vi "Teleop.vi"(10 "Match Info":T1={"Autonomous Elapsed Seconds"=0.0, "TeleOp Elapsed Seconds"=0.0, "Disabled Elapsed Seconds"=0.0, "Visited Autonomous"=FALSE, "Visited TeleOp"=FALSE, "Visited Disabled"=FALSE, "Autonomous Settings"={"Autonomous Style"=enum."Independent", "VI Refnum"=refnum}}, 11 "Call Context":T2) -> ()   [LabVIEW 2011]
doc: "This VI is called for each TeleOp packet received from the DS where the robot is not disabled. It is often used to read from the joysticks and update I/O or to update setpoints for timed control loops. It should complete and return within 20 milliseconds or it may miss DS packets."
uses:
  <vilib>/Rock Robotics/WPI/DriverStation/WPI_DriverStationDerivedRobotMode.ctl
  <vilib>/Rock Robotics/WPI/DriverStation/WPI_DriverStationMatch Info.ctl
  Robot Global Data.vi
  <vilib>/Rock Robotics/WPI/Solenoid/Deprecated/WPI_SolenoidSetBool.vi
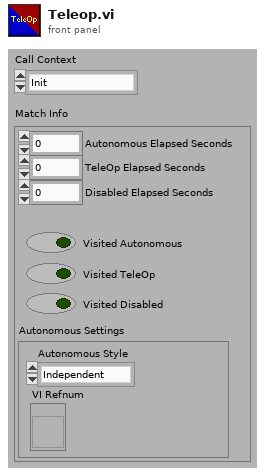
[diagram p1: front panel]
types:
  T1 = typedef "WPI_DriverStationMatch Info.ctl" = cluster{"Autonomous Elapsed Seconds":dbl, "TeleOp Elapsed Seconds":dbl, "Disabled Elapsed Seconds":dbl, "Visited Autonomous":bool, "Visited TeleOp":bool, "Visited Disabled":bool, "Autonomous Settings":cluster{"Autonomous Style":enum16{"Iterative", "Independent"}, "VI Refnum":refnum<vi>}}
  T2 = typedef "WPI_DriverStationDerivedRobotMode.ctl" = enum16{"Init", "Execute", "Stop"}
  T3 = typedef "WPI_DigitalInputDevRef.ctl" = cluster{"DevStatus":errorcluster, "DIO Channel":T4, "Digital Module":T5}
  T4 = typedef "FPGA_DIOChannel.ctl" = enum8{"DIO 1", "DIO 2", "DIO 3", "DIO 4", "DIO 5", "DIO 6", "DIO 7", "DIO 8", "DIO 9", "DIO 10", "DIO 11", "DIO 12", "DIO 13", "DIO 14", "Invalid"}
  T5 = typedef "FPGA_TypedefDigitalModule.ctl" = enum16{"Digital Module 1", "Digital Module 2"}
  T6 = typedef "WPI_ServoDeviceRef.ctl" = cluster{"DeviceStatus":errorcluster, "Digital Module":T5, "PWM Channel":T7, "DeadBand":T8}
  T7 = typedef "FPGA_DIOPWMChannel.ctl" = enum8{"PWM 1", "PWM 2", "PWM 3", "PWM 4", "PWM 5", "PWM 6", "PWM 7", "PWM 8", "PWM 9", "PWM 10", "Invalid"}
  T8 = typedef "WPI_PWMDeadband.ctl" = cluster{"Name":string, "maxPositivePwm":i32, "minPositivePwm":i32, "centerPwm":i32, "maxNegativePwm":i32, "minNegativePwm":i32, "angularRange":u16}
  T9 = typedef "WPI_RobotDriveDevRef.ctl" = cluster{"DevStatus":errorcluster, "Motors[]":T10[], "Square Inputs":bool, "Max Output":dbl}
  T10 = typedef "WPI_MotorControlDeviceRef.ctl" = cluster{"DeviceStatus":errorcluster, "Type":enum16{"PWM", "CAN"}, "PWM":cluster{"Digital Module":T5, "PWM Channel":T7, "DeadBand":T8}, "CAN":cluster{"Device Number":u8, "Control Mode":T11, "Semaphore":T12, "Max Vout":dbl}, "Invert":bool, "TransformRef":T13, "InvTransformRef":T13}
  T11 = typedef "WPI_CANJaguar_ControlMode.ctl" = enum8{"Percent VBus", "Current", "Speed", "Position", "Voltage"}
  T12 = typedef "Semaphore RefNum" = refnum<k1>
  T13 = typedef "WPI_PWMTransform_ConPane.ctl" = refnum<vi>
  T14 = typedef "WPI_JoystickDevRef.ctl" = cluster{"Device":T15}
  T15 = typedef "WPI_JoystickDeviceEnum.ctl" = enum16{"USB 1", "USB 2", "USB 3", "USB 4", "Kinect 1", "Kinect 2"}
  T16 = typedef "WPI_JoystickButtonState.ctl" = cluster{"Button 1":bool, "Button 2":bool, "Button 3":bool, "Button 4":bool, "Button 5":bool, "Button 6":bool, "Button 7":bool, "Button 8":bool, "Button 9":bool, "Button 10":bool, "Button 11":bool, "Button 12":bool}
  T17 = cluster{"axis 1 (x)":dbl, "axis 2 (y)":dbl, "axis 3 (throttle)":dbl, "axis 4":dbl, "axis 5":dbl, "axis 6":dbl}
  T18 = typedef "WPI_EncoderDevRef.ctl" = cluster{"DevStatus":errorcluster, "EncoderIndex":T19, "CounterIndex":T20, "DistancePerCount":dbl, "Decoding Type":T21}
  T19 = typedef "FPGA_EncoderIdx.ctl" = enum8{"Enc 0", "Enc 1", "Enc 2", "Enc 3", "Invalid"}
  T20 = typedef "FPGA_CounterCtrSystemIndex.ctl" = enum8{"Ctr 0", "Ctr 1", "Ctr 2", "Ctr 3", "Ctr 4", "Ctr 5", "Ctr 6", "Ctr 7", "Invalid"}
  T21 = typedef "WPI_EncoderType.ctl" = enum16{"1x", "2x", "4x"}
  T22 = typedef "WPI_SolenoidDevRef.ctl" = cluster{"DevStatus":errorcluster, "Solenoid Module":T23, "Forward Solenoid Channel":T24, "Reverse Solenoid Channel":T24}
  T23 = typedef "FPGA_TypedefSolenoidModule.ctl" = enum16{"Solenoid Module 1", "Solenoid Module 2"}
  T24 = typedef "WPI_SolenoidChannel.ctl" = enum8{"Solenoid 1", "Solenoid 2", "Solenoid 3", "Solenoid 4", "Solenoid 5", "Solenoid 6", "Solenoid 7", "Solenoid 8", "Invalid"}
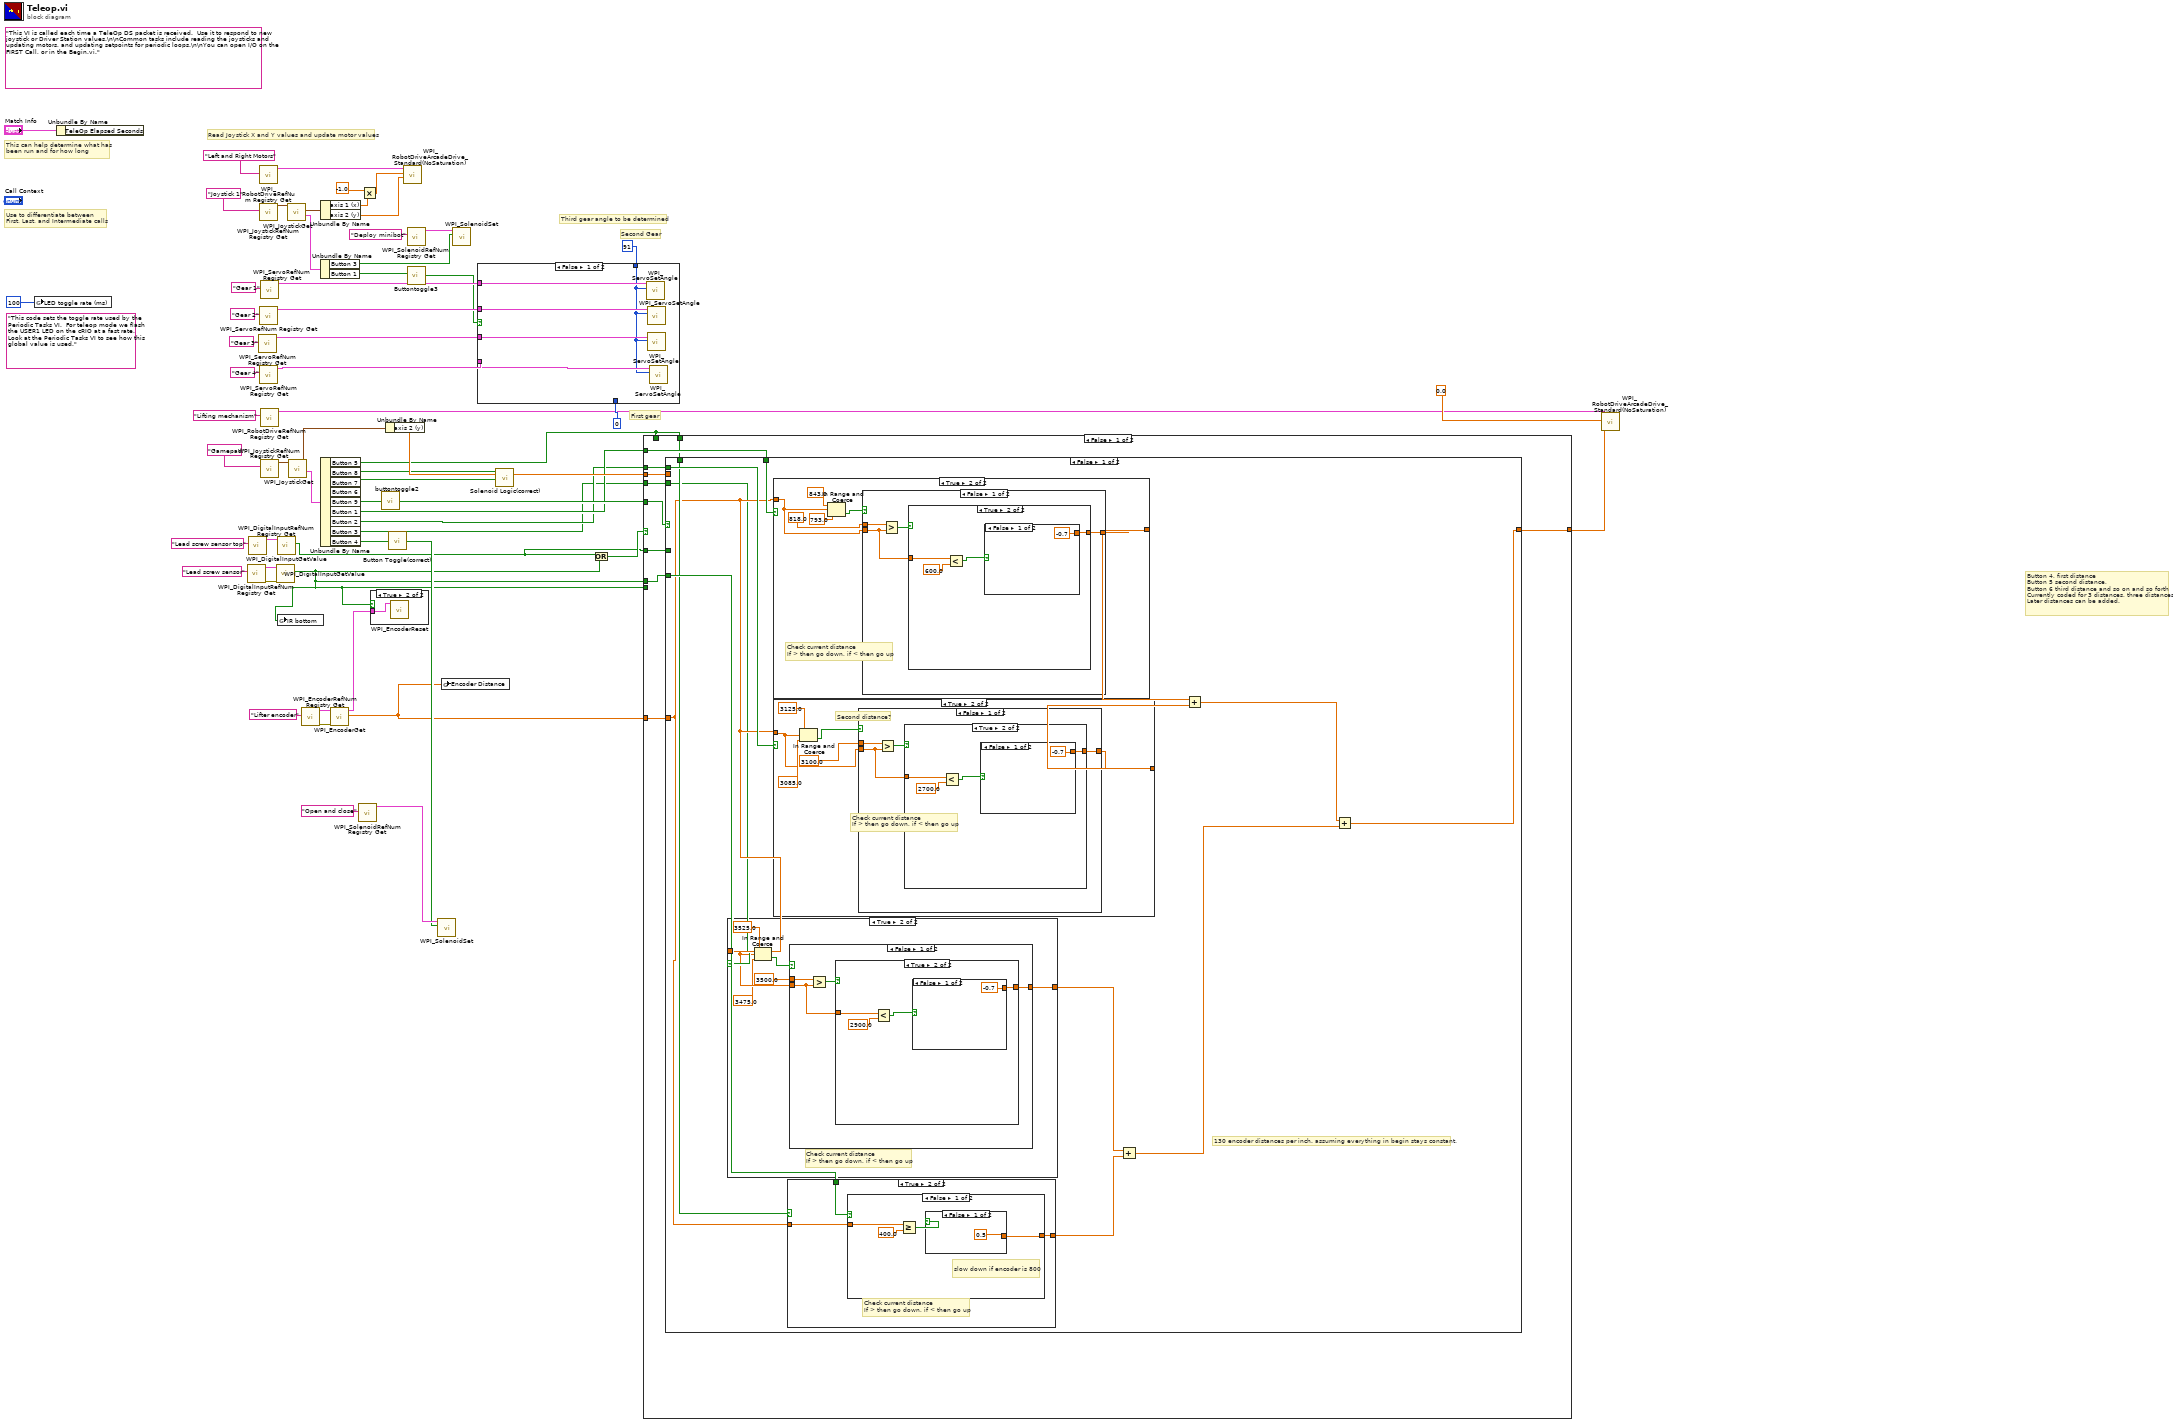
[diagram p0: block diagram]
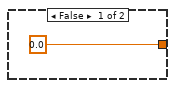
[diagram p3: hidden frame]
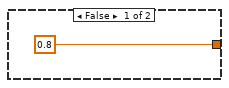
[diagram p4: hidden frame]
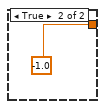
[diagram p5: hidden frame]
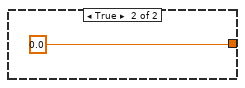
[diagram p6: hidden frame]
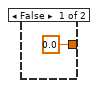
[diagram p7: hidden frame]
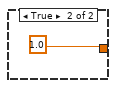
[diagram p8: hidden frame]
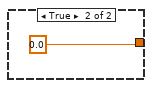
[diagram p9: hidden frame]
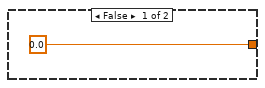
[diagram p10: hidden frame]
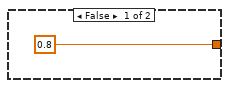
[diagram p11: hidden frame]
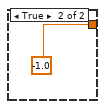
[diagram p12: hidden frame]
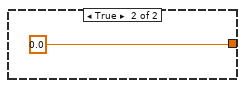
[diagram p13: hidden frame]
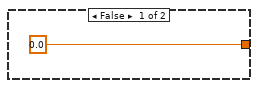
[diagram p14: hidden frame]
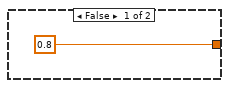
[diagram p15: hidden frame]
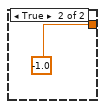
[diagram p16: hidden frame]
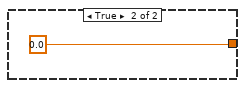
[diagram p17: hidden frame]
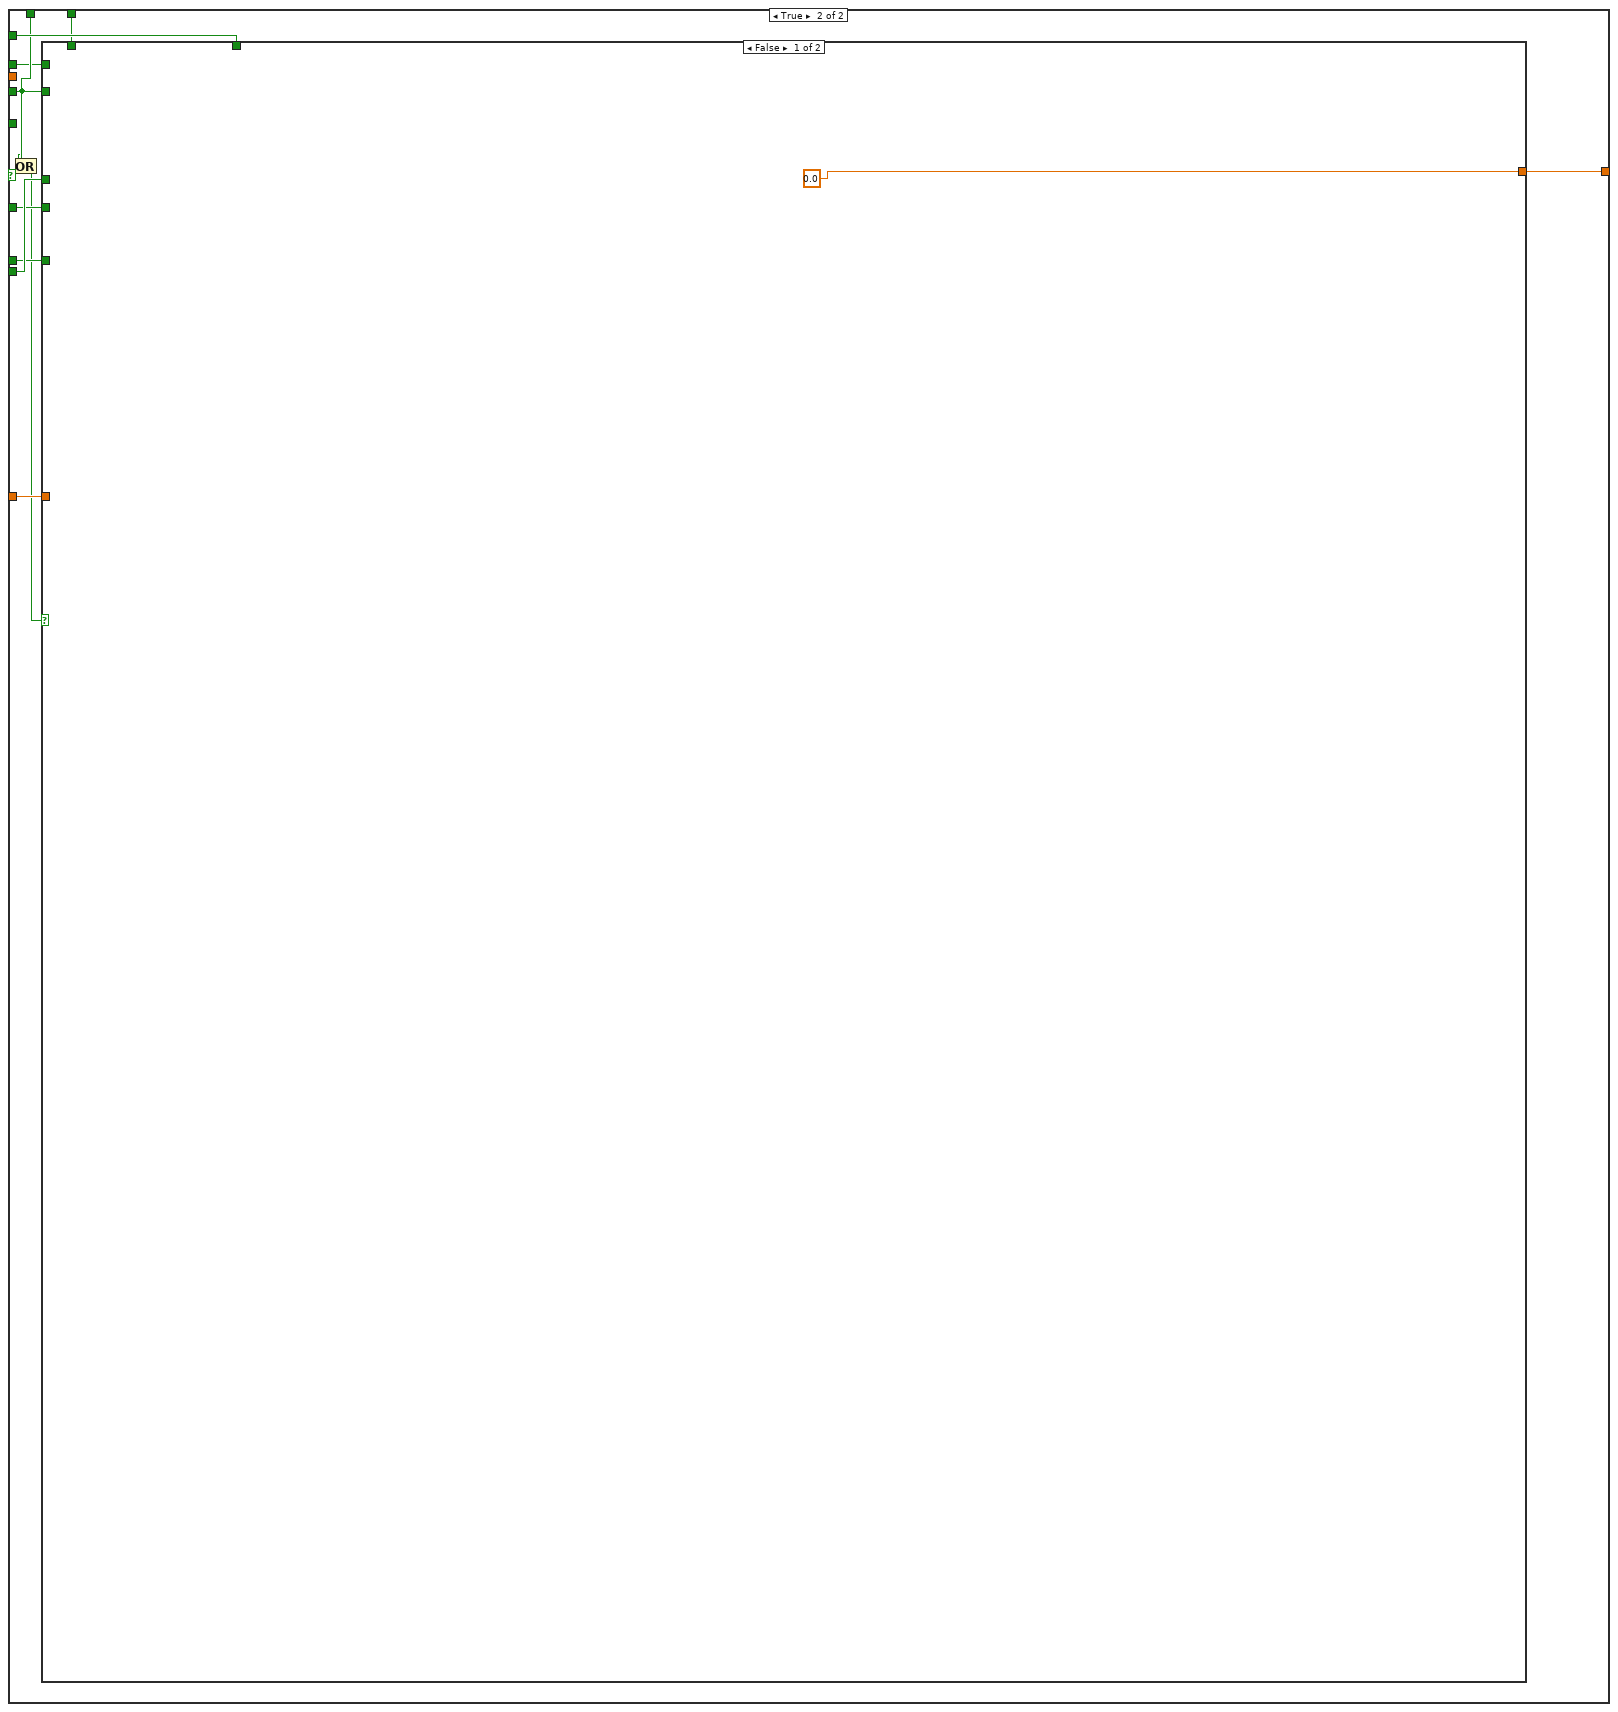
[diagram p19: hidden frame]
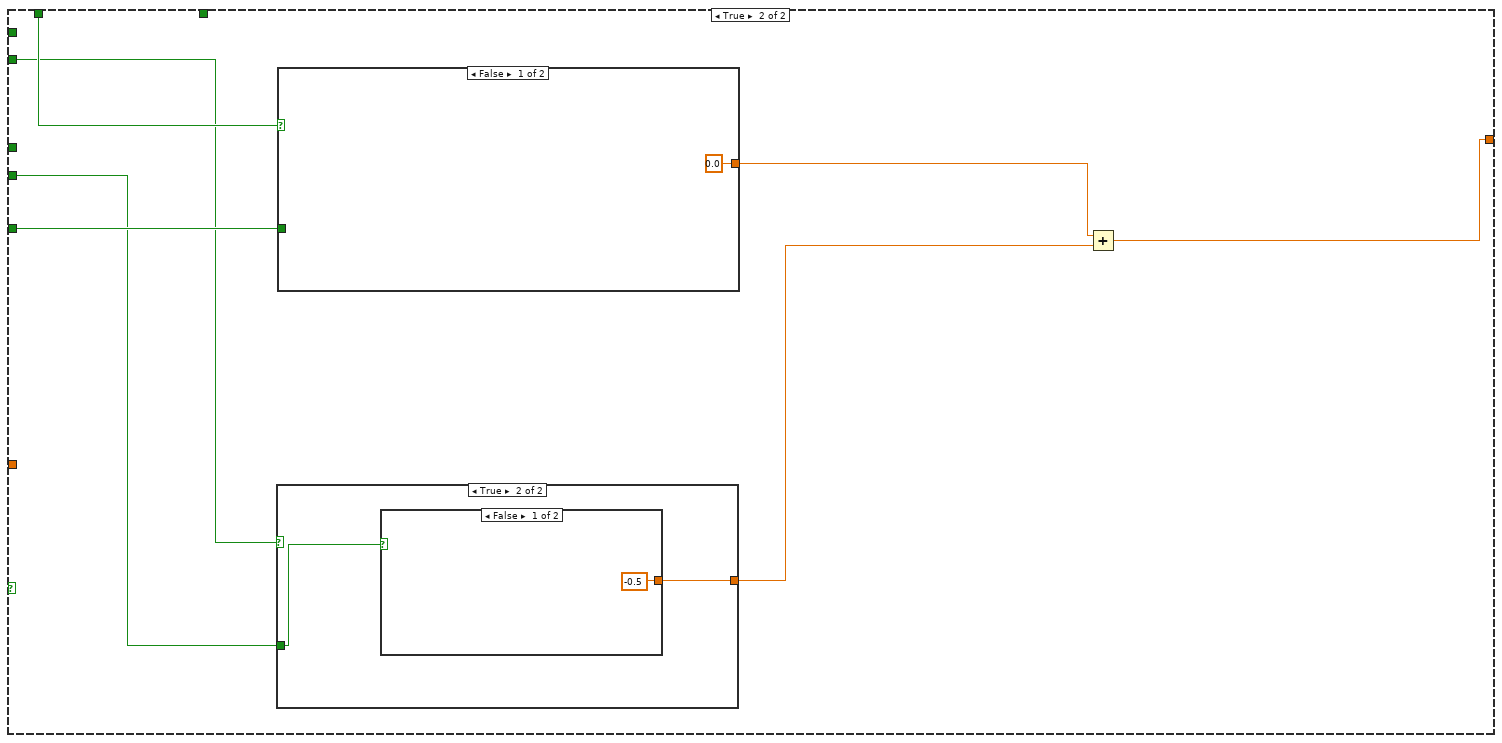
[diagram p20: hidden frame]
diagram:
  (unwired) "This code sets the toggle rate used by the Periodic Tasks VI.  For teleop mode we flash the USER1 LED on the cRIO at a fast rate.  Look at the Periodic Tasks VI to see how this global value is used."
  (unwired) "This VI is called each time a TeleOp DS packet is received.  Use it to respond to new joystick or Driver Station values.\n\nCommon tasks include reading the joysticks and updating motors, and updating setpoints for periodic loops.\n\nYou can open I/O on the FIRST Call, or in the Begin.vi."
  # "First gear"
  # "Button 4, first distance\nButton 5 second distance,\nButton 6 third distance and so on and so forth\nCurrently coded for 3 distances, three distances. Later distances can be added."
  # "Third gear angle to be determined"
  # "Second Gear"
  # "Use to differentiate between\nFirst, Last, and Intermediate calls"
  # "This can help determine what has\nbeen run and for how long"
  # "Read Joystick X and Y values and update motor values"
  n1 = global write "Robot Global Data.vi" "LED toggle rate (ms)"(u32 100 ("LED ms toggle rate")) -> ()
  n2 = Unbundle By Name("Match Info") -> ()  [unwired: 1 out]
  n3 = call <vilib>:"WPI_DigitalInputRefNum Registry Get.vi"("refnum name"="Lead screw sensor") -> ("error out"=w37:errorcluster, "DigitalInputDevRef"=w34:T3)  [unwired: 1 in, 8 out]
  n4 = call <vilib>:"WPI_DigitalInputRefNum Registry Get.vi"("refnum name"="Lead screw sensor top") -> ("DigitalInputDevRef"=w35:T3)  [unwired: 1 in, 9 out]
  n5 = call <vilib>:"WPI_ServoRefNum Registry Get.vi"("refnum name"="Gear 3") -> ("ServoDeviceRef"=w48:T6)  [unwired: 1 in, 9 out]
  n6 = call <vilib>:"WPI_RobotDriveRefNum Registry Get.vi"("refnum name"="Left and Right Motors") -> ("RobotDriveDevRef"=w59:T9)  [unwired: 1 in, 9 out]
  n7 = call <vilib>:"WPI_JoystickRefNum Registry Get.vi"("refnum name"="Joystick 1") -> ("JoystickDevRef"=w54:T14)  [unwired: 1 in, 9 out]
  n8 = call <vilib>:"WPI_ServoRefNum Registry Get.vi"("refnum name"="Gear 2") -> ("ServoDeviceRef"=w47:T6)  [unwired: 1 in, 9 out]
  n9 = call <vilib>:"WPI_ServoRefNum Registry Get.vi"("refnum name"="Gear 4") -> ("ServoDeviceRef"=w49:T6)  [unwired: 1 in, 9 out]
  n10 = call <vilib>:"WPI_ServoRefNum Registry Get.vi"("refnum name"="Gear 1") -> ("ServoDeviceRef"=w46:T6)  [unwired: 1 in, 9 out]
  n11 = call <vilib>:"WPI_RobotDriveRefNum Registry Get.vi"("refnum name"="Lifting mechanism") -> ("RobotDriveDevRef"=w26:T9)  [unwired: 1 in, 9 out]
  n12 = call <vilib>:"WPI_JoystickRefNum Registry Get.vi"("refnum name"="Gamepad") -> ("JoystickDevRef"=w41:T14)  [unwired: 1 in, 9 out]
  n13 = call <vilib>:"WPI_DigitalInputGetValue.vi"("error in (no error)"=w37, "DigitalInputDevRef"=w34) -> ("Value"=w1:bool)  [unwired: 9 out]
  n14 = call <vilib>:"WPI_DigitalInputGetValue.vi"("DigitalInputDevRef"=w35) -> ("Value"=w6:bool)  [unwired: 1 in, 9 out]
  n15 = global write "Robot Global Data.vi" "IR bottom"(w1) -> ()
  n16 = call <vilib>:"WPI_JoystickGet.vi"("JoystickDevRef"=w54) -> ("Buttons"=w43:T16, "Axes"=w58:T17)  [unwired: 1 in, 4 out]
  n17 = call <vilib>:"WPI_JoystickGet.vi"("JoystickDevRef"=w41) -> ("Buttons"=w42:T16, "Axes"=w39:T17)  [unwired: 1 in, 4 out]
  n18 = call <vilib>:"WPI_EncoderRefNum Registry Get.vi"("refnum name"="Lifter encoder") -> ("error out"=w29:errorcluster, "EncoderDevRef"=w28:T18)  [unwired: 1 in, 8 out]
  n19 = Unbundle By Name(w43) -> ("Button 3"=w3:bool, "Button 1"=w17:bool)
  n20 = Unbundle By Name(w58) -> ("axis 1 (x)"=w22:dbl, "axis 2 (y)"=w57:dbl)
  n21 = Unbundle By Name(w42) -> ("Button 5"=w7:bool, "Button 8"=w8:bool, "Button 7"=w9:bool, "Button 9"=w15:bool, "Button 1"=w13:bool, "Button 2"=w12:bool, "Button 3"=w11:bool, "Button 4"=w19:bool)  [unwired: 1 out]
  n22 = call <vilib>:"WPI_EncoderGet.vi"("error in (no error)"=w29, "EncoderDevRef"=w28) -> ("Distance"=w2:dbl, "EncoderDevRef"=w25:T18)  [unwired: 8 out]
  n23 = call <vilib>:"WPI_SolenoidRefNum Registry Get.vi"("refnum name"="Open and close") -> ("SolenoidDevRef"=w23:T22)  [unwired: 1 in, 9 out]
  n24 = Multiply(x=-1.0, y=w22) -> (x*y=w20:dbl)
  n25 = case shown="True" w1 {
    tunnel: w25 -> [_ w62]
    frame False {
    }
    frame True {
      n26 = call <vilib>:"WPI_EncoderReset.vi"("EncoderDevRef"=w62) -> ()  [unwired: 1 in, 10 out]
    }
  }
  n27 = call "buttontoggle2.vi"("Button Input"=w15) -> ("Toggled output"=w14:bool)
  n28 = Unbundle By Name(w39) -> ("axis 2 (y)"=w27:dbl)
  n29 = call "Button Toggle(correct).vi"("Button Input"=w19) -> ("Toggled output"=w18:bool)
  n30 = call <vilib>:"WPI_RobotDriveArcadeDrive_Standard(NoSaturation).vi"("Y axis value"=w57, "X axis value"=w20, "RobotDriveDevRef"=w59) -> ()  [unwired: 1 in, 8 out]
  n31 = call <vilib>:"WPI_SolenoidRefNum Registry Get.vi"("refnum name"="Deploy minibot") -> ("SolenoidDevRef"=w4:T22)  [unwired: 1 in, 9 out]
  n32 = call "Buttontoggle3.vi"("Button Input"=w17) -> ("Boolean"=w16:bool)
  n33 = call-poly <vilib>:"WPI_SolenoidSet.vi"("Value"=w18, "SolenoidDevRef"=w23) -> ()  [unwired: 1 in, 9 out]
  n34 = global write "Robot Global Data.vi" "Encoder Distance"(w2) -> ()
  n35 = call-poly <vilib>:"WPI_SolenoidSet.vi"("Value"=w3, "SolenoidDevRef"=w4) -> ()  [unwired: 1 in, 9 out]
  n36 = case shown="False" w16 {
    tunnel: w49 -> [w67 w69]
    tunnel: w48 -> [w66 w70]
    tunnel: w47 -> [w65 w71]
    tunnel: w46 -> [w64 w72]
    tunnel: 91 ("Angle") -> [w63 _]
    tunnel: 0 ("Angle") -> [_ w68]
    frame False {
      n37 = call <vilib>:"WPI_ServoSetAngle.vi"("Angle"=w63, "ServoDeviceRef"=w64) -> ()  [unwired: 1 in, 9 out]
      n38 = call <vilib>:"WPI_ServoSetAngle.vi"("Angle"=w63, "ServoDeviceRef"=w65) -> ()  [unwired: 1 in, 9 out]
      n39 = call <vilib>:"WPI_ServoSetAngle.vi"("Angle"=w63, "ServoDeviceRef"=w66) -> ()  [unwired: 1 in, 9 out]
      n40 = call <vilib>:"WPI_ServoSetAngle.vi"("Angle"=w63, "ServoDeviceRef"=w67) -> ()  [unwired: 1 in, 9 out]
    }
    frame True {
      n41 = call <vilib>:"WPI_ServoSetAngle.vi"("Angle"=w68, "ServoDeviceRef"=w70) -> ()  [unwired: 1 in, 9 out]
      n42 = call <vilib>:"WPI_ServoSetAngle.vi"("Angle"=w68, "ServoDeviceRef"=w69) -> ()  [unwired: 1 in, 9 out]
      n43 = call <vilib>:"WPI_ServoSetAngle.vi"("Angle"=w68, "ServoDeviceRef"=w72) -> ()  [unwired: 1 in, 9 out]
      n44 = call <vilib>:"WPI_ServoSetAngle.vi"("Angle"=w68, "ServoDeviceRef"=w71) -> ()  [unwired: 1 in, 9 out]
    }
  }
  n45 = call "Solenoid Logic(correct)"("Button 7"=w9, "Button 8"=w8) -> ()  [unwired: 1 in]
  n46 = Or(x=w6, y=w1) -> (x .or. y?=w32:bool)
  n47 = case shown="False" w32 {
    tunnel: w27 -> [w82 _]
    tunnel: w1 -> [_ w175]
    tunnel: [w81 w173] -> w10
    tunnel: w2 -> [w80 w174]
    tunnel: w6 -> [w79 w169]
    tunnel: w14 -> [w78 _]
    tunnel: w13 -> [w77 w172]
    tunnel: w12 -> [w76 w167]
    tunnel: w11 -> [w75 w165]
    tunnel: w1 -> [w74 w171]
    tunnel: w7 -> [w73 w170]
    tunnel: w7 -> [_ w168]
    frame False {
      n48 = case shown="False" w78 {
        tunnel: w82 -> [_ w164]
        tunnel: [w86 w164] -> w81
        tunnel: w80 -> [w85 _]
        tunnel: w79 -> [_ _]
        tunnel: w77 -> [w95 _]
        tunnel: w76 -> [w94 _]
        tunnel: w75 -> [w84 _]
        tunnel: w74 -> [w93 _]
        tunnel: w73 -> [w92 _]
        frame False {
          # "130 encoder distances per inch. assuming everything in begin stays constant."
          n49 = case shown="True" w84 {
            tunnel: w85 -> [_ w99]
            tunnel: [0.0 ("Y axis value") w101] -> w83
            frame False {
            }
            frame True {
              # "Check current distance\nIf > then go down, if < then go up"
              n50 = In Range and Coerce(upper limit=3525.0, x=w99, lower limit=3475.0) -> (In Range?=w100:bool)  [unwired: 1 out]
              n51 = case shown="False" w100 {
                tunnel: 3500.0 ("y") -> [w106 _]
                tunnel: w99 -> [w103 _]
                tunnel: [w104 0.0 ("Y axis value")] -> w101
                frame False {
                  n52 = Greater?(x=w106, y=w103) -> (0:w105:bool)
                  n53 = case shown="True" w105 {
                    tunnel: [0.8 ("Y axis value") w111] -> w104
                    tunnel: w103 -> [_ w110]
                    frame False {
                    }
                    frame True {
                      n54 = Less?(x=w110, y=2900.0) -> (x < y?=w108:bool)
                      n55 = case shown="False" w108 {
                        tunnel: [-0.7 ("Y axis value") -1.0 ("Y axis value")] -> w111
                        frame False {
                        }
                        frame True {
                        }
                      }
                    }
                  }
                }
                frame True {
                }
              }
            }
          }
          n56 = case shown="True" w94 {
            tunnel: w85 -> [_ w128]
            tunnel: [0.0 ("Y axis value") w127] -> w89
            frame False {
            }
            frame True {
              # "Check current distance\nIf > then go down, if < then go up"
              # "Second distance?"
              n57 = In Range and Coerce(upper limit=3125.0, x=w128, lower limit=3085.0) -> (In Range?=w130:bool)  [unwired: 1 out]
              n58 = case shown="False" w130 {
                tunnel: 3100.0 ("y") -> [w136 _]
                tunnel: w128 -> [w133 _]
                tunnel: [w134 0.0 ("Y axis value")] -> w127
                frame False {
                  n59 = Greater?(x=w136, y=w133) -> (0:w135:bool)
                  n60 = case shown="True" w135 {
                    tunnel: [0.8 ("Y axis value") w141] -> w134
                    tunnel: w133 -> [_ w140]
                    frame False {
                    }
                    frame True {
                      n61 = Less?(x=w140, y=2700.0) -> (x < y?=w138:bool)
                      n62 = case shown="False" w138 {
                        tunnel: [-0.7 ("Y axis value") -1.0 ("Y axis value")] -> w141
                        frame False {
                        }
                        frame True {
                        }
                      }
                    }
                  }
                }
                frame True {
                }
              }
            }
          }
          n63 = case shown="True" w95 {
            tunnel: w85 -> [_ w149]
            tunnel: [0.0 ("Output") w147] -> w90
            frame False {
            }
            frame True {
              # "Check current distance\nIf > then go down, if < then go up"
              n64 = In Range and Coerce(upper limit=843.0, x=w149, lower limit=793.0) -> (In Range?=w146:bool)  [unwired: 1 out]
              n65 = case shown="False" w146 {
                tunnel: 818.0 ("y") -> [w155 _]
                tunnel: w149 -> [w152 _]
                tunnel: [w153 0.0 ("Y axis value")] -> w147
                frame False {
                  n66 = Greater?(x=w155, y=w152) -> (0:w154:bool)
                  n67 = case shown="True" w154 {
                    tunnel: [0.8 ("Y axis value") w160] -> w153
                    tunnel: w152 -> [_ w159]
                    frame False {
                    }
                    frame True {
                      n68 = Less?(x=w159, y=600.0) -> (x < y?=w157:bool)
                      n69 = case shown="False" w157 {
                        tunnel: [-0.7 ("Y axis value") -1.0 ("Y axis value")] -> w160
                        frame False {
                        }
                        frame True {
                        }
                      }
                    }
                  }
                }
                frame True {
                }
              }
            }
          }
          n70 = case shown="True" w92 {
            tunnel: [0.0 ("Y axis value") w118] -> w91
            tunnel: w93 -> [_ w117]
            tunnel: w85 -> [_ w116]
            frame False {
            }
            frame True {
              # "Check current distance\nIf > then go down, if < then go up"
              n71 = case shown="False" w117 {
                tunnel: [w119 0.0 ("Y axis value")] -> w118
                tunnel: w116 -> [w120 _]
                frame False {
                  # "slow down if encoder is 800"
                  n72 = Greater Or Equal?(x=w120, y=400.0) -> (x >= y?=w121:bool)
                  n73 = case shown="False" w121 {
                    tunnel: [0.5 ("Y axis value") 1.0 ("Y axis value")] -> w119
                    frame False {
                    }
                    frame True {
                    }
                  }
                }
                frame True {
                }
              }
            }
          }
          n74 = Add(x=w83, y=w91) -> (x+y=w87:dbl)
          n75 = Add(x=w90, y=w89) -> (x+y=w88:dbl)
          n76 = Add(x=w88, y=w87) -> (x+y=w86:dbl)
        }
        frame True {
        }
      }
    }
    frame True {
      n77 = Or(x=w168, y=w165) -> (x .or. y?=w166:bool)
      n78 = case shown="False" w166 {
        tunnel: w175 -> [_ _]
        tunnel: [0.0 ("Y axis value") w177] -> w173
        tunnel: w174 -> [_ _]
        tunnel: w172 -> [_ _]
        tunnel: w167 -> [_ _]
        tunnel: w165 -> [_ w180]
        tunnel: w171 -> [_ w182]
        tunnel: w170 -> [_ w183]
        tunnel: w169 -> [_ w181]
        frame False {
        }
        frame True {
          n79 = case shown="True" w180 {
            tunnel: [0.0 ("Y axis value") w186] -> w178
            tunnel: w181 -> [_ w185]
            frame False {
            }
            frame True {
              n80 = case shown="False" w185 {
                tunnel: [-0.5 ("Y axis value") 0.0 ("Y axis value")] -> w186
                frame False {
                }
                frame True {
                }
              }
            }
          }
          n81 = case shown="False" w183 {
            tunnel: [0.0 ("Y axis value") w191] -> w179
            tunnel: w182 -> [_ w190]
            frame False {
            }
            frame True {
              n82 = case shown="False" w190 {
                tunnel: [0.5 ("Y axis value") 0.0 ("Y axis value")] -> w191
                frame False {
                }
                frame True {
                }
              }
            }
          }
          n83 = Add(x=w179, y=w178) -> (x+y=w177:dbl)
        }
      }
    }
  }
  n84 = call <vilib>:"WPI_RobotDriveArcadeDrive_Standard(NoSaturation).vi"("Y axis value"=w10, "X axis value"=0.0, "RobotDriveDevRef"=w26) -> ()  [unwired: 1 in, 8 out]
